vi "LV to ITX  Retrieve.vi"(0 "File or Folder Path":path=path "C:/", 1 "Data Type":T1=enum."DAT", 2 "DAT header length":i32=11, 5 "offset":i32, 7 "length":i32=1, 9 "index":T2={"A"=1, "B"=0, "C"=2, "D"=0, "E"=3, "N1"=0, "N2"=0, "N3"=0, "N4"=0}, 11 "error in (no error)":errorcluster) -> (4 "A vs B":cluster{dbl[], dbl[]}[](graph), 6 "C vs D":cluster{dbl[], dbl[]}[](graph), 8 "E":dbl[][](graph), 10 "N":cluster{"N1":dbl, "N2":dbl, "N3":dbl, "N4":dbl}={"N1"=0.0624995231628418, "N2"=0.0624995231628418, "N3"=0.0624995231628418, "N4"=0.0624995231628418} {"N4" format="%#_6p"; "N3" format="%#_6p"; "N2" format="%#_6p"; "N1" format="%#_6p"}, 14 "Notes":string)   [LabVIEW 2019, in "Data.ITX.lvclass"]
uses:
  Data.ITX.lvclass
  graph_utilities/src/graph_utilities.lvclass
  Data/Data.lvclass
  <vilib>/Utility/miscctls.llb/LVOffsetAndMultiplierTypeDef.ctl
  Typedefs/Retrieve Data Type.ctl
panel:
  in  "D  is time?":bool
  in  "B is time?":bool
  out "time":string[][](table)
  in  "Use Folder Index File?":bool
  in  "Generate Folder Index File?":bool
  in  "Ez name":string="Ez name"
  in  "Ey name":string="Ey name"
  in  "Ex name":string="Ex name"
  in  "C y name":string="C y name"
  in  "D x name":string="D x name"
  in  "A y name":string="A y name"
  in  "B x name":string="B x name"
  out "Index, Wavenames":string[][](table)
  in  "recolor traces?":bool
  in  "Ex":T3={"Offset"=0.0, "Multiplier"=1.0}
  in  "Ey":T3={"Offset"=0.0, "Multiplier"=1.0}
  out "Path":path
  out "counter":i32
  out "pattern":string="*.dat"
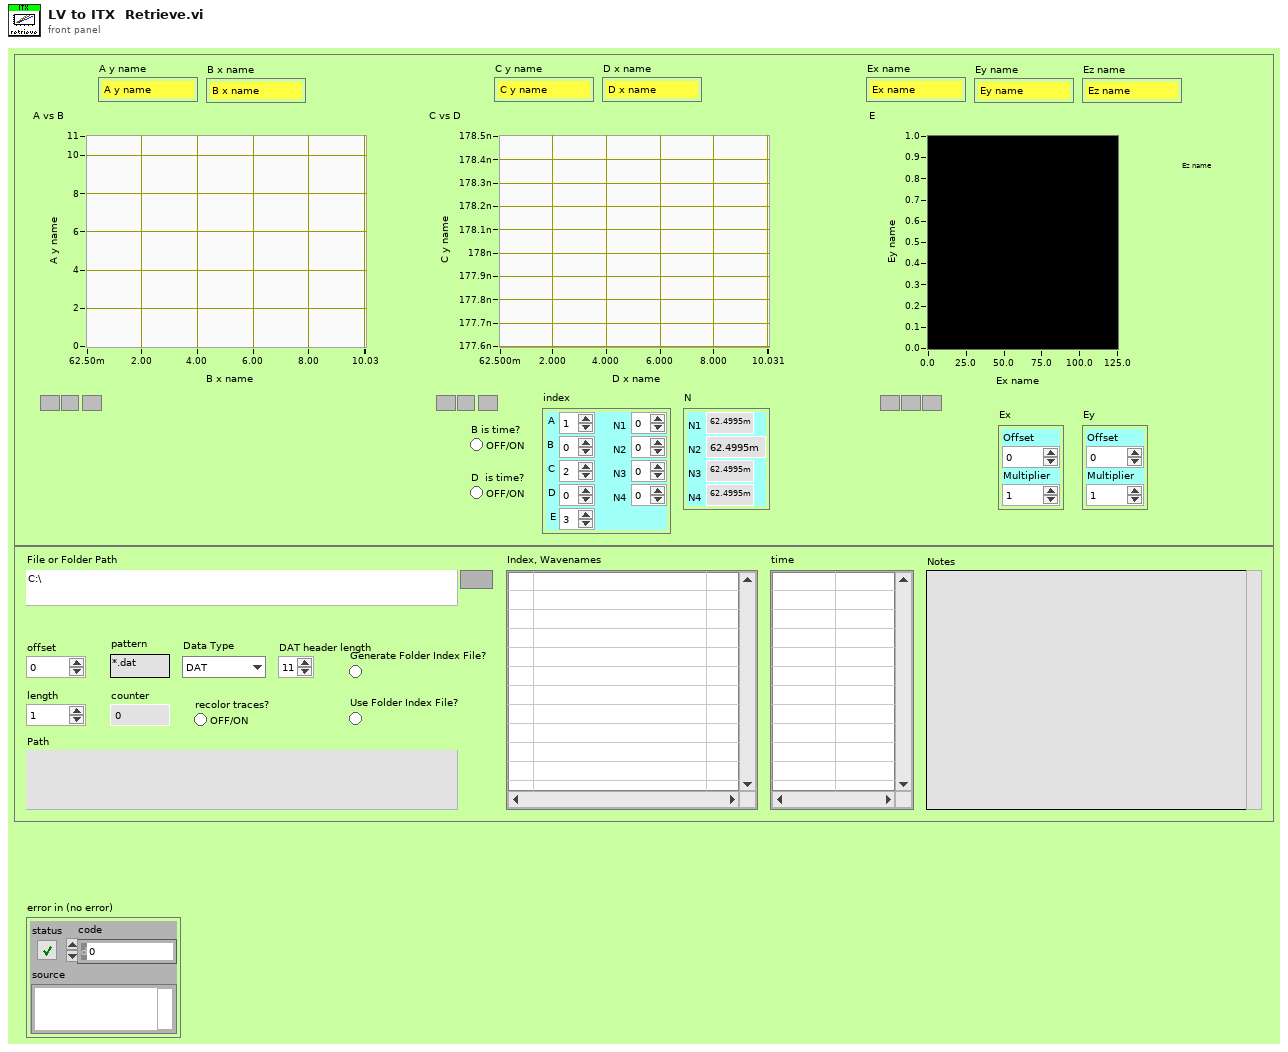
[diagram p1: front panel]
types:
  T1 = typedef "Data.ITX.lvclass/Retrieve Data Type.ctl" = enum16{"ITX", "ITX w/ 2D", "DAT", "TDMS"}
  T2 = cluster{"A":i32, "B":i32, "C":i32, "D":i32, "E":i32, "N1":i32, "N2":i32, "N3":i32, "N4":i32}
  T3 = typedef "LVOffsetAndMultiplierTypeDef.ctl" = cluster{"Offset":dbl, "Multiplier":dbl}
  T4 = typedef "Data.lvclass/Dictionary--cluster.ctl" = cluster{"key":string, "value":variant}
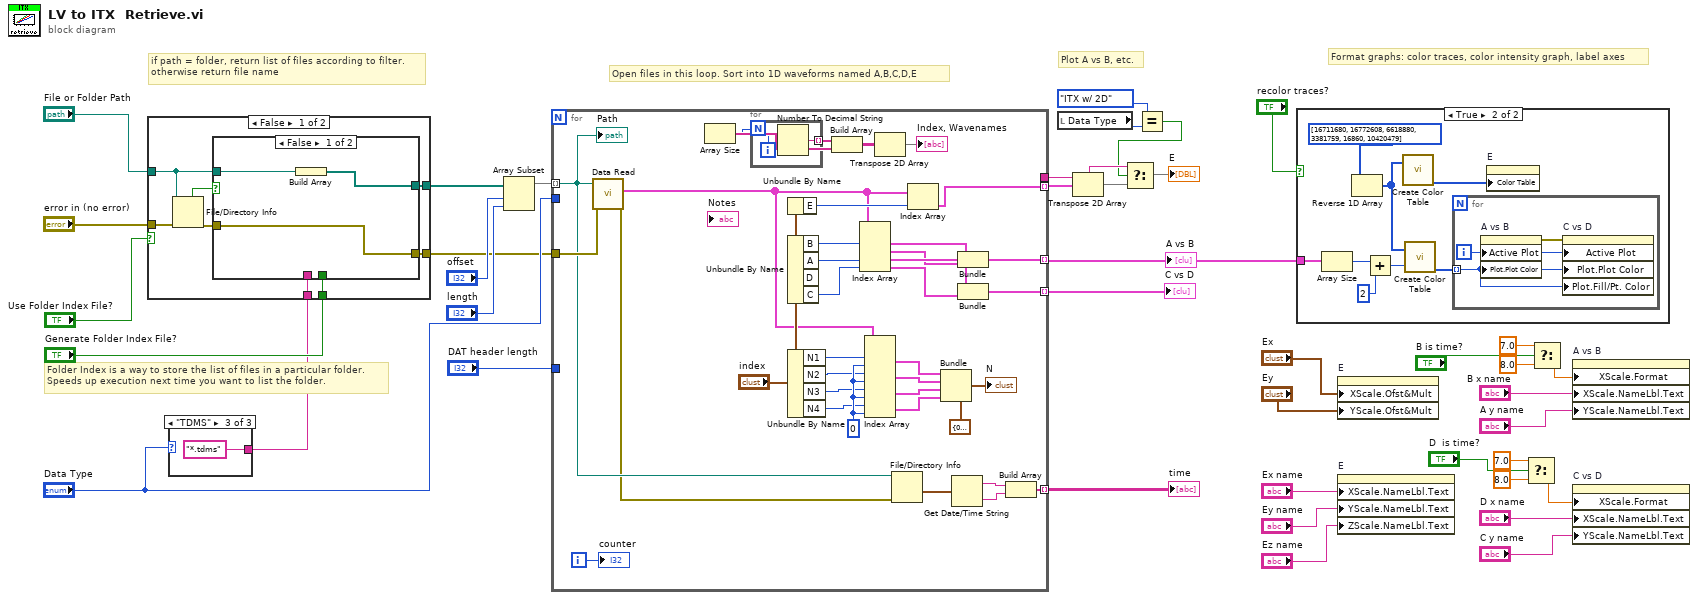
[diagram p0: block diagram]
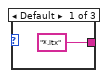
[diagram p2: hidden frame]
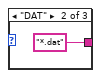
[diagram p3: hidden frame]
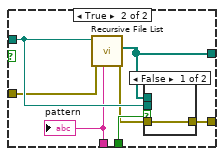
[diagram p5: hidden frame]
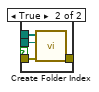
[diagram p6: hidden frame]
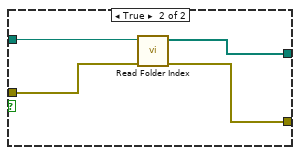
[diagram p7: hidden frame]
diagram:
  # "Plot A vs B, etc."
  # "Format graphs: color traces, color intensity graph, label axes"
  # "Open files in this loop. Sort into 1D waveforms named A,B,C,D,E"
  # "Folder Index is a way to store the list of files in a particular folder.\nSpeeds up execution next time you want to list the folder."
  # "if path = folder, return list of files according to filter.\notherwise return file name"
  n1 = case shown="\"TDMS\"" "Data Type" {
    tunnel: ["*.itx" ("pattern") "*.dat" ("pattern") "*.tdms" ("pattern")] -> w4
    frame Default {
    }
    frame "DAT" {
    }
    frame "TDMS" {
    }
  }
  n2 = case shown="False" "Use Folder Index File?" {
    tunnel: [w49 w69] -> w38
    tunnel: "File or Folder Path" -> [w51 w70]
    tunnel: "Generate Folder Index File?" -> [w48 _]
    tunnel: w4 -> [w47 _]
    tunnel: "error in (no error)" -> [w46 w68]
    tunnel: [w44 w67] -> w1
    frame False {
      n3 = File/Directory Info(path=w51, error in=w46) -> (directory=w50:bool, error out=w45:errorcluster)  [unwired: 5 out]
      n4 = case shown="False" w50 {
        tunnel: [w54 w60] -> w49
        tunnel: w51 -> [w53 w61]
        tunnel: w48 -> [_ w58]
        tunnel: w47 -> [_ w59]
        tunnel: w45 -> [w52 w56]
        tunnel: [w52 w57] -> w44
        frame False {
          n5 = Build Array(w53) -> (w54:path[])
        }
        frame True {
          n6 = call <vilib>:"Recursive File List.vi"("pattern"=w59, "error in (no error)"=w56, "Folder Path"=w61) -> ("error out"=w55:errorcluster, "All Files in Dir"=w60:path[])  [unwired: 4 in, 3 out]
          n7 = case shown="False" w58 {
            tunnel: w60 -> [_ w66]
            tunnel: w61 -> [_ w65]
            tunnel: w55 -> [w62 w64]
            tunnel: [w62 w63] -> w57
            frame False {
            }
            frame True {
              n8 = call "Create Folder Index.vi"("error in (no error)"=w64, "File or Folder Path"=w65, "All Files in Dir"=w66) -> ("error out"=w63:errorcluster)  [unwired: 8 in]
            }
          }
          "pattern" <- w59
        }
      }
    }
    frame True {
      n9 = call "Read Folder Index.vi"("error in (no error)"=w68, "File or Folder Path"=w70) -> ("error out"=w67:errorcluster, "Files"=w69:path[])  [unwired: 8 in]
    }
  }
  n10 = Array Subset(array=w38, index="offset", length="length") -> (w17:path[])
  n11 = for {
    tunnel: w17 -> [w73] mode=indexing
    tunnel: [w108] -> w29 mode=indexing
    tunnel: [w107] -> w28 mode=indexing
    tunnel: [w86] -> w33 mode=indexing
    tunnel: [w100] -> w31
    tunnel: [w79] -> w20 mode=indexing
    tunnel: "Data Type" -> [_]
    tunnel: "DAT header length" -> [_]
    tunnel: w1 -> [w74]
    i -> [w110]
    w99 = 0 ("disabled index (col)")
    n12 = call "Data Read.vi"("error in (no error)"=w74, "path"=w73) -> ("error out"=w72:errorcluster, "Data (Dictionary)"=w71:T4[])  [unwired: 6 in, 2 out]
    n13 = Unbundle By Name("index") -> ("E"=w91:i32)
    n14 = Unbundle By Name("index") -> ("B"=w90:i32, "A"=w89:i32, "D"=w88:i32, "C"=w87:i32)
    n15 = Unbundle By Name("index") -> ("N1"=w92:i32, "N2"=w93:i32, "N3"=w94:i32, "N4"=w95:i32)
    n16 = Index Array(array=w71, index #1=w90, index #2=w89, index #3=w88, index #4=w87) -> (element #1=w84:T4, element #2=w83:T4, element #3=w103:T4, element #4=w106:T4)
    n17 = Index Array(array=w71, index (row) #1=w92, index (col) #1=w99, index (row) #2=w93, index (col) #2=w99, index (row) #3=w94, index (col) #3=w99, index (row) #4=w95, index (col) #4=w99) -> (element #1=w80:T4, element #2=w81:T4, element #3=w82:T4, element #4=w98:T4)
    n18 = File/Directory Info(path=w73, error in=w72) -> (last mod=w78:timestamp)  [unwired: 6 out]
    n19 = Index Array(array=w71, index=w91) -> (element=w86:T4)
    n20 = Bundle(cluster=cluster{"N1":dbl, "N2":dbl, "N3":dbl, "N4":dbl} {"N1"=0.0, "N2"=0.0, "N3"=0.0, "N4"=0.0}, "N1"=w80, "N2"=w81, "N3"=w82, "N4"=w98) -> (→"N":cluster{"N1":dbl, "N2":dbl, "N3":dbl, "N4":dbl})
    n21 = Get Date/Time String(seconds (now)=w78) -> (date string=w76:string, time string=w77:string)  [unwired: 2 in]
    n22 = Bundle("key-value"=w84, "key-value"=w83) -> (w108:cluster{"key-value":T4, "key-value":T4})  [unwired: 1 in]
    n23 = Bundle("key-value"=w103, "key-value"=w106) -> (w107:cluster{"key-value":T4, "key-value":T4})  [unwired: 1 in]
    n24 = Build Array(w76, w77) -> (w79:string[])
    n25 = Array Size(array=w101) -> (size(s)=w75:i32)
    n26 = for {
      N: w75 -> [_]
      tunnel: [w111] -> w105 mode=indexing
      i -> [w112]
      n27 = Number To Decimal String(number=w112) -> (decimal integer string=w111:string)  [unwired: 1 in]
    }
    n28 = Build Array(w105) -> (w102:string[][], w101:string[])
    n29 = Transpose 2D Array(2D array=w102) -> (transposed array=→"Index, Wavenames":string[][])
    "counter" <- w110
    "Path" <- w73
  }
  "A vs B" <- w29
  "C vs D" <- w28
  "time" <- w20
  n30 = local read "Data Type"() -> (w7:T1)
  n31 = Transpose 2D Array(2D array=w33) -> (transposed array=w34:T4[][])
  n32 = Equal?(x=enum16{"ITX", "ITX w/ 2D", "DAT"}."ITX w/ 2D" ("Enum"), y=w7) -> (x = y?=w5:bool)
  n33 = Select(t=w31, s=w5, f=w34) -> (s? t:f=→"E":T4[][])
  n34 = case shown="True" "recolor traces?" {
    tunnel: w29 -> [_ w115]
    frame False {
    }
    frame True {
      n35 = Array Size(array=w115) -> (size(s)=w116:i32)
      n36 = Reverse 1D Array(array=u32[] [16711680, 16772608, 6618880, 3381759, 16860, 10420479] ("color scale")) -> (reversed array=w114:u32[])
      n37 = Add(x=w116, y=2 ("x")) -> (x+y=w120:i32)
      n38 = call "Create Color Table.vi"("Colors []"=w114) -> ("Color Tbl"=w118:u32[])  [unwired: 1 in, 3 out]
      n39 = call "Create Color Table.vi"("Colors []"=w114, "Size (256)"=w120) -> ("Color Tbl"=w117:u32[])  [unwired: 3 out]
      n40 = for {
        tunnel: w117 -> [w121] mode=indexing
        i -> [w122]
        n41 = property on="A vs B" class="XYGraph (strict)"("Active Plot"=w122, "Plot.Plot Color"=w121) -> (error out=w123:errorcluster)  [unwired: 2 in, 1 out]
        n42 = property on="C vs D" class="XYGraph (strict)"(error in=w123, "Active Plot"=w122, "Plot.Plot Color"=w121, "Plot.Fill/Pt. Color"=w121) -> ()  [unwired: 1 in, 2 out]
      }
      n43 = property on="E" class="IntGraph (strict)"("Color Table"=w118) -> ()  [unwired: 2 in, 2 out]
    }
  }
  n44 = property on="E" class="IntGraph (strict)"("XScale.Ofst&Mult"="Ex", "YScale.Ofst&Mult"="Ey") -> ()  [unwired: 2 in, 2 out]
  n45 = property on="E" class="IntGraph (strict)"("XScale.NameLbl.Text"="Ex name", "YScale.NameLbl.Text"="Ey name", "ZScale.NameLbl.Text"="Ez name") -> ()  [unwired: 2 in, 2 out]
  n46 = Select(t=7.0, s="D  is time?", f=8.0) -> (s? t:f=w13:dbl)
  n47 = Select(t=7.0, s="B is time?", f=8.0) -> (s? t:f=w14:dbl)
  n48 = property on="A vs B" class="XYGraph (strict)"("XScale.Format"=w14, "XScale.NameLbl.Text"="B x name", "YScale.NameLbl.Text"="A y name") -> ()  [unwired: 2 in, 2 out]
  n49 = property on="C vs D" class="XYGraph (strict)"("XScale.Format"=w13, "XScale.NameLbl.Text"="D x name", "YScale.NameLbl.Text"="C y name") -> ()  [unwired: 2 in, 2 out]
